vi "save_state.vi"(0 "state":u16(ring) items=["none", "walking", "bicycling", "stairs up"], 2 "peaks":dbl[][](array[numeric])) -> ()   [LabVIEW 2009]
uses:
  activity_info.vi
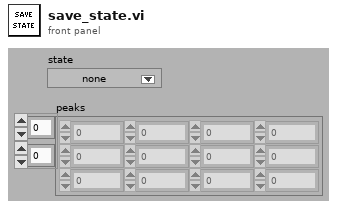
[diagram p1: front panel]
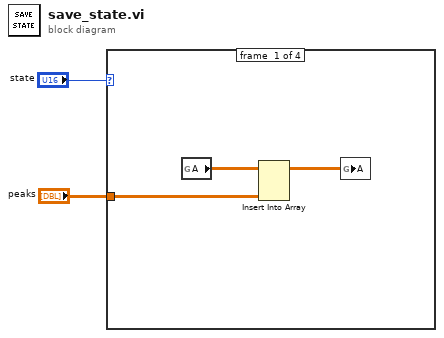
[diagram p0: block diagram]
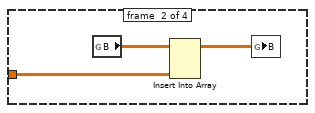
[diagram p2: hidden frame]
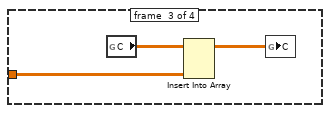
[diagram p3: hidden frame]
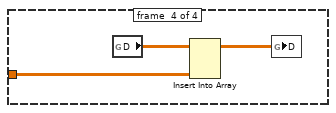
[diagram p4: hidden frame]
diagram:
  n1 = case shown="0, Default" "state" {
    tunnel: "peaks" -> [w5 w6 w9 w12]
    frame #0 {
      n2 = global read "activity_info.vi" "A"() -> (w4:dbl[][])
      n3 = Insert Into Array(array=w4, new element=w5) -> (w3:dbl[][])  [unwired: 2 in]
      n4 = global write "activity_info.vi" "A"(w3) -> ()
    }
    frame #1 {
      n5 = global read "activity_info.vi" "B"() -> (w8:dbl[][])
      n6 = Insert Into Array(array=w8, new element=w6) -> (w7:dbl[][])  [unwired: 2 in]
      n7 = global write "activity_info.vi" "B"(w7) -> ()
    }
    frame #2 {
      n8 = global read "activity_info.vi" "C"() -> (w11:dbl[][])
      n9 = Insert Into Array(array=w11, new element=w9) -> (w10:dbl[][])  [unwired: 2 in]
      n10 = global write "activity_info.vi" "C"(w10) -> ()
    }
    frame #3 {
      n11 = global read "activity_info.vi" "D"() -> (w14:dbl[][])
      n12 = Insert Into Array(array=w14, new element=w12) -> (w13:dbl[][])  [unwired: 2 in]
      n13 = global write "activity_info.vi" "D"(w13) -> ()
    }
  }
